vi "Protocol FG.vi"(7 "Action":T1, 8 "error in (no error)":errorcluster, 10 "Protocol":string(combo), 11 "Device Item Ref in":T2 format="%.0x") -> (0 "error out":errorcluster, 2 "Protocol out":string(combo), 3 "Item Ref out":T2 format="%.0x")   [LabVIEW 2013, in "Instrument Addon Shared.lvlib"]
uses:
  Instrument Addon Shared.lvlib
  <vilib>/NI Veristand/Custom Device API/Custom Device Item Ref.ctl
  Types/FG Control.ctl
  Constants.vi
  <vilib>/NI Veristand/Custom Device API/Get Item Property (String).vi
  <vilib>/NI Veristand/Custom Device API/Set Item Property (String).vi
  <vilib>/NI Veristand/Custom Device API/Custom Device API.lvlib
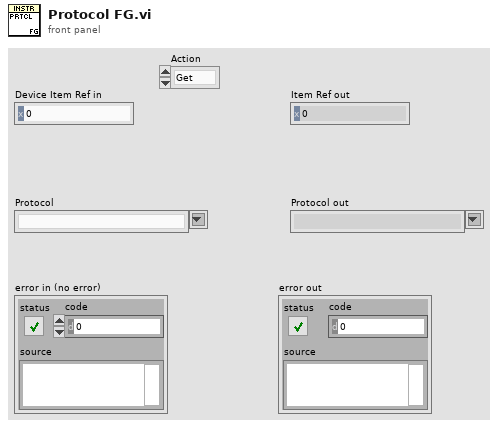
[diagram p1: front panel]
types:
  T1 = typedef "Instrument Addon Shared.lvlib/FG Control.ctl" = enum16{"Get", "Set"}
  T2 = typedef "Custom Device API.lvlib/Custom Device Item Ref.ctl" = u64
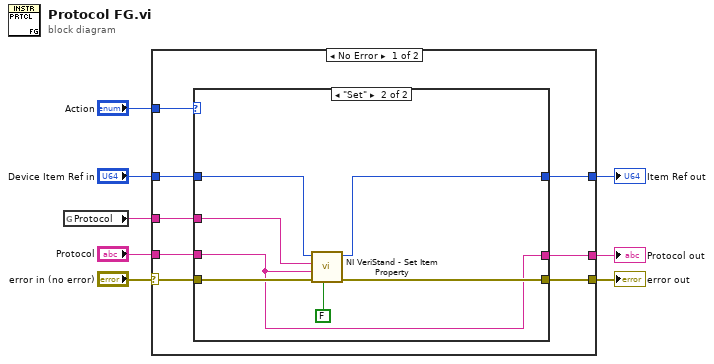
[diagram p0: block diagram]
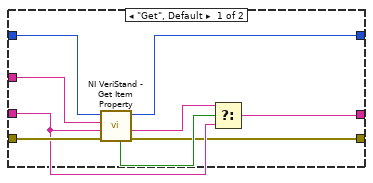
[diagram p2: hidden frame]
diagram:
  n1 = global read "Constants.vi" "Protocol"() -> (w8:string)
  n2 = case shown="No Error" "error in (no error)" {
    selector: "error in (no error)" -> [w11 w35]
    tunnel: w8 -> [w16 _]
    tunnel: [w15 w33] -> w7
    tunnel: "Device Item Ref in" -> [w14 w33]
    tunnel: "Protocol" -> [w13 w34]
    tunnel: [w12 w35] -> w4
    tunnel: [w10 w34] -> w2
    tunnel: "Action" -> [w9 _]
    frame No Error {
      n3 = case shown="\"Set\"" w9 {
        tunnel: w16 -> [w22 w32]
        tunnel: [w23 w31] -> w15
        tunnel: w14 -> [w24 w30]
        tunnel: w13 -> [w19 w27]
        tunnel: [w18 w29] -> w12
        tunnel: w11 -> [w25 w28]
        tunnel: [w17 w27] -> w10
        frame "Get", Default {
          n4 = call-poly <vilib>:"NI VeriStand - Get Item Property.vi"("error in (no error)"=w25, "Default Value"=w19, "Property Name"=w22, "Item Ref in"=w24) -> ("error out"=w18:errorcluster, "Value"=w20:string, "Item Ref out"=w23:T2, "Found?"=w21:bool)  [unwired: 4 in]
          n5 = Select(t=w20, s=w21, f=w19) -> (s? t:f=w17:string)
        }
        frame "Set" {
          n6 = call-poly <vilib>:"NI VeriStand - Set Item Property.vi"("Binary String (T)"=FALSE, "error in (no error)"=w28, "Value"=w27, "Property Name"=w32, "Item Ref in"=w30) -> ("error out"=w29:errorcluster, "Item Ref out"=w31:T2)  [unwired: 4 in, 1 out]
        }
      }
    }
    frame Error {
    }
  }
  "Item Ref out" <- w7
  "error out" <- w4
  "Protocol out" <- w2
